vi "Main.vi"(11 "Module Admin":refnum<class "Delacor_lib_QMH_Module Admin.lvclass">) -> ()   [LabVIEW 2020, in "Launcher.lvlib"]
doc: "This template is based off of the Queued Message Handler design pattern and the Queued Message Handler project template that ships with LabVIEW.\n\nThe main difference is that the queue is private to this module and communication between modules is performed via Broadcast and Request events.\n\nRequest events are wrapped in public API methods and are handled in the Event Handling Loop (EHL) of this VI. Any module can register for Broadcast events sent by this module. The EHL generates messages based on user interface actions.\n\nThe Message Handling Loop (MHL) processes messages generated by the EHL, or by other messages. The messages are string values, so new messages can be added easily to the Message Cases case structure in the MHL. Each message cluster can also provide an optional value for Message Data, which is a variant that can be converted to whatever message-specific data is required.\n_____\nBased on Delacor QMH Project Template 5.0.0.82."
uses:
  Launcher.lvlib
  <vilib>/Delacor/Delacor QMH/Libraries/Module Admin_class/Delacor_lib_QMH_Module Admin.lvclass
  Module Data--cluster.ctl
  Stop Argument--cluster.ctl
  <vilib>/Delacor/Delacor QMH/Libraries/Message Queue_class/Delacor_lib_QMH_Message Queue.lvclass/Delacor_lib_QMH_Message Queue.ctl
  <vilib>/Delacor/Delacor QMH/Libraries/Module Admin_class/Delacor_lib_QMH_Module Admin.lvclass/Delacor_lib_QMH_Module Admin.ctl
  NXP LPCXpresso54608/NXP LPCXpresso54608.lvclass
  NXP LPCXpresso54608/NXP LPCXpresso54608.lvclass/NXP LPCXpresso54608.ctl
  Cypress CY8CKIT-059/Cypress CY8CKIT-059.lvclass
  Cypress CY8CKIT-059/Cypress CY8CKIT-059.lvclass/Cypress CY8CKIT-059.ctl
  Simulated Device/Simulated Device.lvclass
  <vilib>/Utility/miscctls.llb/LVPointTypeDef.ctl
  <vilib>/Delacor/Delacor QMH/Libraries/Message Queue_class/Delacor_lib_QMH_Enqueue Message (Single).vi
  <vilib>/Delacor/Delacor QMH/Libraries/Module Admin_class/Delacor_lib_QMH_Get External Launch.vi
  NXP LPCXpresso54608/Write Serial Port.vi
  Cypress CY8CKIT-059/Write Serial Port.vi
  <vilib>/Utility/error.llb/Error Cluster From Error Code.vi
  <vilib>/ErrorRing/Error Ring.xnode
  <vilib>/Delacor/Delacor QMH/Libraries/Message Queue_class/Delacor_lib_QMH_Message Queue.lvclass
  Hardware Interface/Hardware Interface.lvlib
panel:
  in  "Serial Port":refnum<visa-resource-name>
  in  "Device":enum16{"NXP", "Cypress", "Simulada"}(ring)
  in  "Open":bool
  out "error out":errorcluster
  out "Status":string
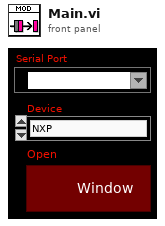
[diagram p1: front panel]
types:
  T1 = typedef "Launcher.lvlib/Request Events--cluster.ctl" = cluster{"Stop Module":refnum<user-event>, "Show Panel":refnum<user-event>, "Hide Panel":refnum<user-event>, "Get Module Execution Status":refnum<user-event>, "Show Diagram":refnum<user-event>}
  T2 = typedef "Hardware Interface.lvlib/Broadcast Events--cluster.ctl" = cluster{"Module Did Init":refnum<user-event>, "Status Updated":refnum<user-event>, "Error Reported":refnum<user-event>, "Module Did Stop":refnum<user-event>, "Update Module Execution Status":refnum<user-event>}
  T3 = typedef "Launcher.lvlib/Module Data--cluster.ctl" = cluster{"Status":string}
  T4 = enum32{"invalid lock state", "Not Locked", "Locked (No Password)", "Password-protected"}
  T5 = typedef "Launcher.lvlib/Stop Argument--cluster.ctl" = cluster{"Origin":string, "Exit via Stop Module Req?":bool, "Wait for Module to stop?":bool}
  T6 = typedef "LVPointTypeDef.ctl" = cluster{"Horizontal":i16, "Vertical":i16}
  T7 = enum32{"Invalid", "Standard", "Closed", "Hidden", "Minimized", "Maximized"}
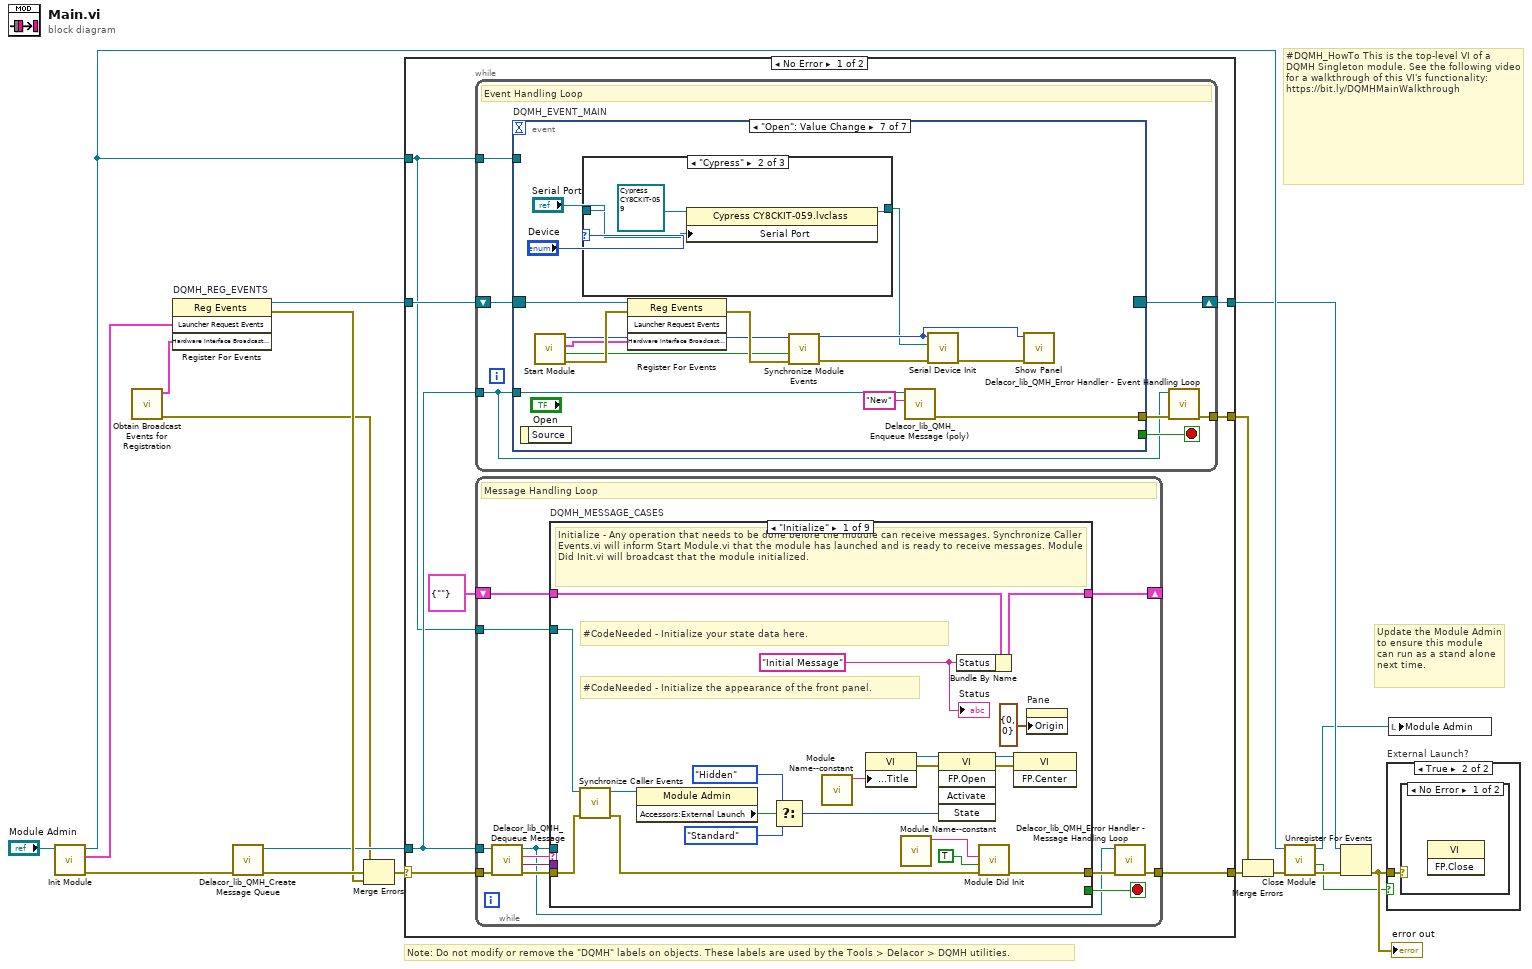
[diagram p0: block diagram]
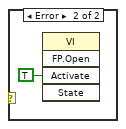
[diagram p3: hidden frame]
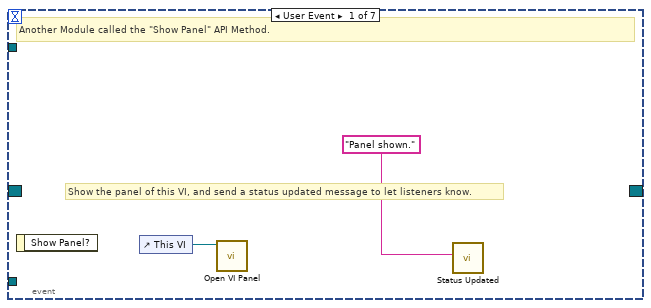
[diagram p4: hidden frame]
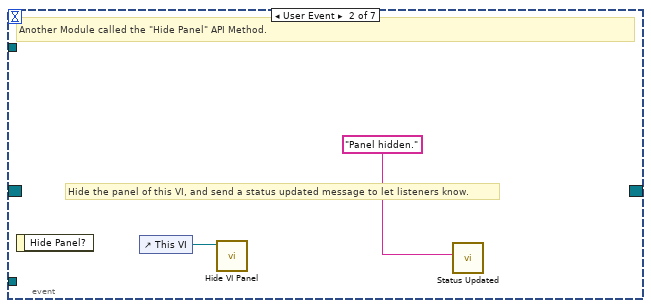
[diagram p5: hidden frame]
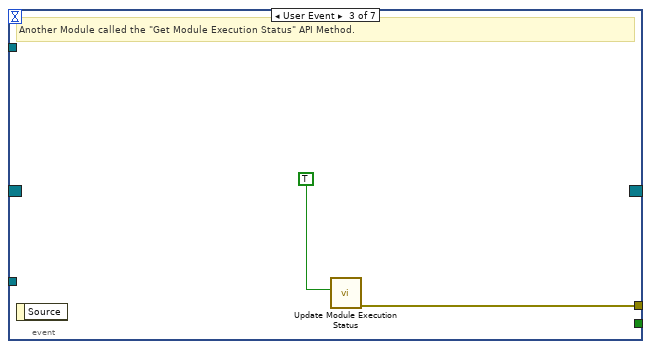
[diagram p6: hidden frame]
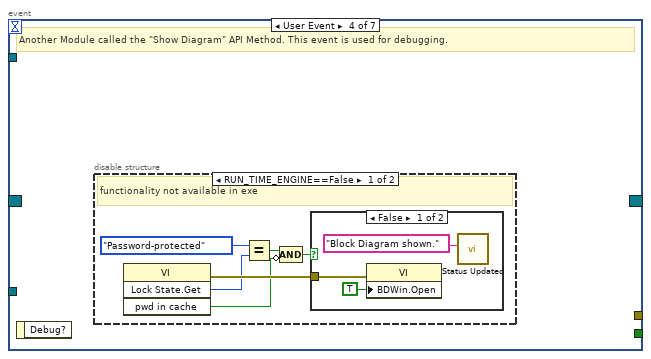
[diagram p7: hidden frame]
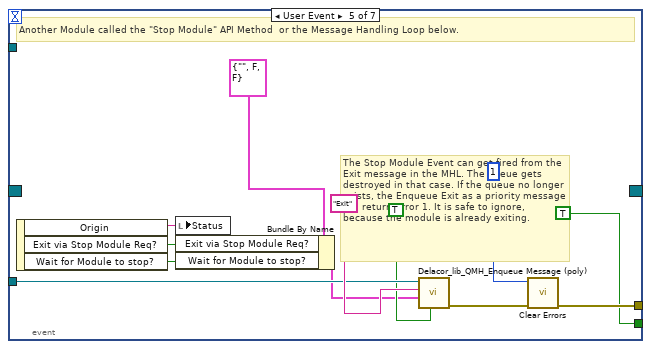
[diagram p10: hidden frame]
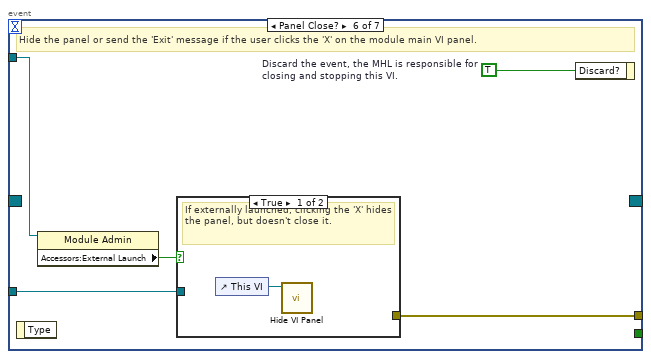
[diagram p11: hidden frame]
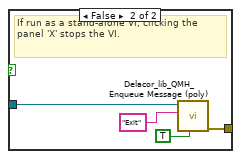
[diagram p12: hidden frame]
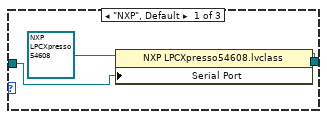
[diagram p13: hidden frame]
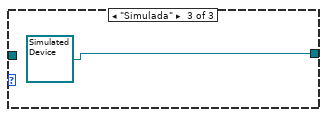
[diagram p14: hidden frame]
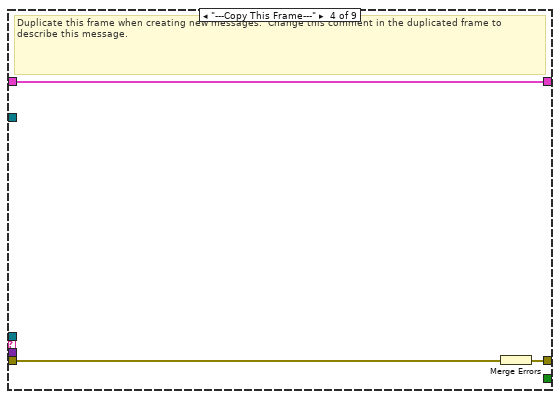
[diagram p17: hidden frame]
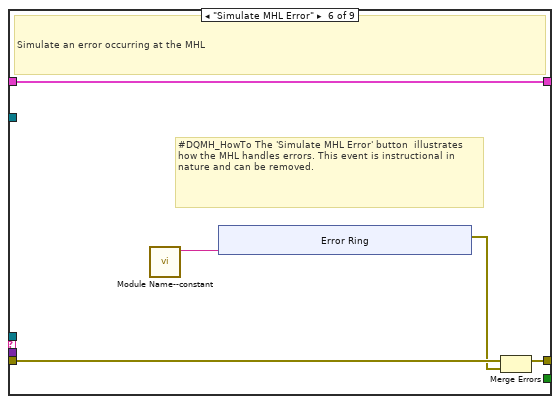
[diagram p19: hidden frame]
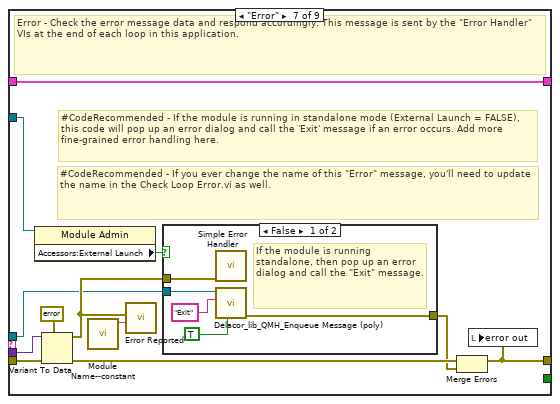
[diagram p20: hidden frame]
diagram:
  # "#DQMH_HowTo This is the top-level VI of a DQMH Singleton module. See the following video for a walkthrough of this VI's functionality: https://bit.ly/DQMHMainWalkthrough"
  # "Note: Do not modify or remove the \"DQMH\" labels on objects. These labels are used by the Tools > Delacor > DQMH utilities."
  # "Update the Module Admin to ensure this module can run as a stand alone next time."
  n1 = call "Init Module.vi"("Singleton Module Admin in"="Module Admin") -> ("error out"=w18:errorcluster, "Launcher Request Events"=w7:T1, "Singleton Module Admin out"=w10:refnum<class "Delacor_lib_QMH_Module Admin.lvclass">)  [unwired: 8 in]
  n2 = call "Obtain Broadcast Events for Registration.vi"() -> ("error out"=w1:errorcluster, "Hardware Interface Broadcast Events"=w2:T2)  [unwired: 9 in, 1 out]
  n3 = register-events "DQMH_REG_EVENTS"(w7, w2) -> (reference out=w8:refnum<event-registration>, error out=w11:errorcluster)  [unwired: 2 in]
  n4 = call <vilib>:"Delacor_lib_QMH_Create Message Queue.vi"("error in (no error)"=w18) -> ("error out"=w13:errorcluster, "Message Queue"=w6:refnum<class "Delacor_lib_QMH_Message Queue.lvclass">)  [unwired: 9 in]
  n5 = Merge Errors(w1, w13, w11) -> (w12:errorcluster)
  n6 = case shown="No Error" w12 {
    selector: w12 -> [w25 w195]
    tunnel: [w27 w194] -> w19
    tunnel: [w24 w200] -> w9
    tunnel: w8 -> [w22 w200]
    tunnel: w6 -> [w21 w193]
    tunnel: [w26 _] -> w16
    tunnel: w10 -> [w20 w196]
    frame No Error {
      n7 = while {
        tunnel: w21 -> [w28]
        shift-right: [w31] -> w24
        shift-left: w22 -> [w32]
        tunnel: [w33] -> w26
        tunnel: w20 -> [w29]
        stop <- w30 stop-if-true
        # "Event Handling Loop"
        n8 = event "DQMH_EVENT_MAIN" shown="[6] \"Open\": Value Change" {
          selector: w32 -> [_ _ _ _ _ _ w79]
          dyn-events: [_ _ _ _ _ _ _] -> w31
          timeout: _ -> [_ _ _ _ _ _ _]
          tunnel: [_ _ _ _ TRUE ("Discard?") _ _] -> w30
          tunnel: w28 -> [_ _ _ _ w57 w64 w85]
          tunnel: [_ _ w40 _ w60 w66 w86] -> w34
          tunnel: w29 -> [_ _ _ _ _ w63 _]
          event User Event {
            # "Show the panel of this VI, and send a status updated message to let listeners know."
            # "Another Module called the \"Show Panel\" API Method."
            n9 = event-data() -> ()  [unwired: 1 in, 1 out]
            n10 = control-ref of="This VI"() -> (w36:refnum<vi>)
            n11 = call "Open VI Panel.vi"("VI"=w36) -> ()  [unwired: 10 in, 1 out]
            n12 = call "Status Updated.vi"("Status"="Panel shown." ("format string")) -> ()  [unwired: 10 in, 1 out]
          }
          event User Event {
            # "Hide the panel of this VI, and send a status updated message to let listeners know."
            # "Another Module called the \"Hide Panel\" API Method."
            n13 = event-data() -> ()  [unwired: 1 in, 1 out]
            n14 = control-ref of="This VI"() -> (w38:refnum<vi>)
            n15 = call "Hide VI Panel.vi"("VI"=w38) -> ()  [unwired: 10 in, 1 out]
            n16 = call "Status Updated.vi"("Status"="Panel hidden." ("format string")) -> ()  [unwired: 10 in, 1 out]
          }
          event User Event {
            # "Another Module called the \"Get Module Execution Status\" API Method."
            n17 = event-data() -> ()  [unwired: 1 in, 1 out]
            n18 = call "Update Module Execution Status.vi"("Running?"=TRUE) -> ("error out"=w40:errorcluster)  [unwired: 10 in]
          }
          event User Event {
            # "Another Module called the \"Show Diagram\" API Method. This event is used for debugging."
            n19 = event-data() -> ()  [unwired: 1 in, 1 out]
            n20 = disable-structure shown="RUN_TIME_ENGINE==False" {
              frame condition #0 (active) {
                # "functionality not available in exe"
                n21 = invoke class="VI" method="Lock State.Get"() -> (error out=w46:errorcluster, "Get Lock State"=w45:T4, "pwd in cache"=w42:bool)  [unwired: 4 in, 1 out]
                n22 = Equal?(x=T4."Password-protected", y=w45) -> (x = y?=w43:bool)
                n23 = Compound Arithmetic op=AND(w43, invert w42) -> (w41:bool)
                n24 = case shown="False" w41 {
                  tunnel: w46 -> [w49 _]
                  frame False {
                    n25 = property class="VI"(error in=w49, "BDWin.Open"=TRUE ("Block Diagram Window:Open")) -> ()  [unwired: 1 in, 2 out]
                    n26 = call "Status Updated.vi"("Status"="Block Diagram shown." ("format string")) -> ()  [unwired: 10 in, 1 out]
                  }
                  frame True {
                    # "Password-protected VI, and the password is not in the cache. Do not show the diagram."
                  }
                }
              }
              frame condition #1 {
              }
            }
          }
          event User Event {
            # "The Stop Module Event can get fired from the Exit message in the MHL. The queue gets destroyed in that case. If the queue no longer exists, the Enqueue Exit as a priority message will return error 1. It is safe to ignore, because the module is already exiting."
            # "Another Module called the \"Stop Module\" API Method  or the Message Handling Loop below."
            n27 = event-data() -> ("Origin"=w56:string, "Exit via Stop Module Req?"=w52:bool, "Wait for Module to stop?"=w51:bool)  [unwired: 1 in]
            n28 = local write "Status"(w56) -> ()
            n29 = Bundle By Name(cluster=T5 {"Origin"="", "Exit via Stop Module Req?"=FALSE, "Wait for Module to stop?"=FALSE} ("Stop Argument"), "Exit via Stop Module Req?"=w52, "Wait for Module to stop?"=w51) -> (w50:T5)
            n30 = call-poly <vilib>:"Delacor_lib_QMH_Enqueue Message (poly).vi"("Priority Message? (F)"=TRUE, "Message Data"=w50, "Message"="Exit", "Message Queue in"=w57) -> ("error out"=w61:errorcluster)  [unwired: 6 in, 1 out]
            n31 = call <vilib>:"Clear Errors.vi"("error in (no error)"=w61, "specific error code to clear (0: all)"=1) -> ("error out"=w60:errorcluster)  [unwired: 4 in, 1 out]
          }
          event Panel Close? {
            w65 = TRUE  # Discard the event, the MHL is responsible for closing and stopping this VI.
            # "Hide the panel or send the 'Exit' message if the user clicks the 'X' on the module main VI panel."
            n32 = event-data() -> ()  [unwired: 1 in, 1 out]
            n33 = property class="Module Admin"(reference=w63) -> ("Accessors:External Launch"=w62:bool)  [unwired: 1 in, 2 out]
            n34 = case shown="True" w62 {
              tunnel: w64 -> [_ w70]
              tunnel: [_ w71] -> w66
              frame True {
                # "If externally launched, clicking the 'X' hides the panel, but doesn't close it."
                n35 = control-ref of="This VI"() -> (w67:refnum<vi>)
                n36 = call "Hide VI Panel.vi"("VI"=w67) -> ()  [unwired: 10 in, 1 out]
              }
              frame False {
                # "If run as a stand-alone VI, clicking the panel 'X' stops the VI."
                n37 = call-poly <vilib>:"Delacor_lib_QMH_Enqueue Message (poly).vi"("Priority Message? (F)"=TRUE, "Message"="Exit", "Message Queue in"=w70) -> ("error out"=w71:errorcluster)  [unwired: 7 in, 1 out]
              }
            }
            n38 = event-data("Discard?"=w65) -> ()  [unwired: 1 in, 1 out]
          }
          event "Open": Value Change {
            n39 = event-data() -> ()  [unwired: 1 in, 1 out]
            n40 = call "Start Module.vi"() -> ("error out"=w82:errorcluster, "Wait for Event Sync?"=w80:bool, "Hardware Interface Broadcast Events"=w78:T2, "Module ID"=w81:i32)  [unwired: 8 in]
            n41 = case shown="\"Cypress\"" "Device" {
              tunnel: [w88 w92 refnum<class "Simulated Device.lvclass"> refnum ("Simulated Device.lvclass")] -> w72
              tunnel: "Serial Port" -> [w87 w90 _]
              frame "NXP", Default {
                n42 = property class="NXP LPCXpresso54608.lvclass"(reference=refnum<class "NXP LPCXpresso54608.lvclass"> refnum ("NXP LPCXpresso54608.lvclass"), "Serial Port"=w87) -> (reference out=w88:refnum<class "NXP LPCXpresso54608.lvclass">)  [unwired: 1 in, 1 out]
              }
              frame "Cypress" {
                n43 = property class="Cypress CY8CKIT-059.lvclass"(reference=refnum<class "Cypress CY8CKIT-059.lvclass"> refnum ("Cypress CY8CKIT-059.lvclass"), "Serial Port"=w90) -> (reference out=w92:refnum<class "Cypress CY8CKIT-059.lvclass">)  [unwired: 1 in, 1 out]
              }
              frame "Simulada" {
              }
            }
            n44 = register-events(reference=w79, error in=w82, w78) -> (error out=w83:errorcluster)  [unwired: 1 in, 1 out]
            n45 = call "Synchronize Module Events.vi"("error in (no error)"=w83, "Wait for Event Sync?"=w80, "Module ID"=w81) -> ("error out"=w77:errorcluster, "Module ID (dup)"=w75:i32)  [unwired: 7 in]
            n46 = call-poly <vilib>:"Delacor_lib_QMH_Enqueue Message (poly).vi"("Message"="New", "Message Queue in"=w85) -> ("error out"=w86:errorcluster)  [unwired: 8 in, 1 out]
            n47 = call "Serial Device Init.vi"("error in (no error)"=w77, "MCU.lvclass"=w72, "Module ID"=w75) -> ("error out"=w76:errorcluster)  [unwired: 8 in]
            n48 = call "Show Panel.vi"("error in (no error)"=w76, "Module ID"=w75) -> ()  [unwired: 9 in, 1 out]
          }
        }
        n49 = call-dynamic "Delacor_lib_QMH_Error Handler - Event Handling Loop.vi"("error in (no error)"=w34, "Message Queue in"=w28) -> ("dup error in"=w33:errorcluster)  [unwired: 8 in, 1 out]
      }
      n50 = while {
        tunnel: w21 -> [w96]
        shift-right: [w100] -> _
        shift-left: T3 {"Status"=""} ("Data Cluster") -> [w101]
        tunnel: w25 -> [w104]
        tunnel: [w102] -> w27
        tunnel: w20 -> [w94]
        stop <- w99 stop-if-true
        # "Message Handling Loop"
        n51 = call-dynamic "Delacor_lib_QMH_Dequeue Message.vi"("error in (no error)"=w104, "Message Queue in"=w96) -> ("error out"=w103:errorcluster, "Message Data"=w97:variant, "Message"=w98:string, "Message Queue out"=w95:refnum<class "Delacor_lib_QMH_Message Queue.lvclass">)  [unwired: 6 in]
        n52 = case "DQMH_MESSAGE_CASES" shown="\"Initialize\"" w98 {
          selector: w98 -> [_ _ _ _ _ _ _ _ w180]
          tunnel: w95 -> [_ _ _ _ _ _ w150 w172 _]
          tunnel: w103 -> [w123 w127 w129 w132 w134 w139 w157 w178 w182]
          tunnel: [w121 w127 w129 w131 w134 w138 w153 w175 w183] -> w105
          tunnel: w101 -> [w112 w126 w128 w130 w133 w136 w152 w171 w181]
          tunnel: [w111 w126 w128 w130 w133 w136 w152 w171 w181] -> w100
          tunnel: [_ _ _ _ _ _ _ w170 _] -> w99
          tunnel: w97 -> [_ _ _ _ _ _ w151 w169 _]
          tunnel: w94 -> [w113 _ _ _ _ _ w149 w164 _]
          frame "Initialize" {
            w106 = "Initial Message" ("Initial Message")
            # "#CodeNeeded - Initialize the appearance of the front panel."
            # "#CodeNeeded - Initialize your state data here."
            # "Initialize - Any operation that needs to be done before the module can receive messages. Synchronize Caller Events.vi will inform Start Module.vi that the module has launched and is ready to receive messages. Module Did Init.vi will broadcast that the module initialized."
            n53 = call "Synchronize Caller Events.vi"("error in (no error)"=w123, "Singleton Module Admin in"=w113) -> ("error out"=w122:errorcluster, "Singleton Module Admin out"=w108:refnum<class "Delacor_lib_QMH_Module Admin.lvclass">)  [unwired: 8 in]
            n54 = property class="Module Admin"(reference=w108) -> ("Accessors:External Launch"=w117:bool)  [unwired: 1 in, 2 out]
            n55 = Select(t=T7."Hidden" ("State"), s=w117, f=T7."Standard" ("State")) -> (s? t:f=w114:T7)
            n56 = call "Module Name--constant.vi"() -> ("Module Name"=w120:string)  [unwired: 11 in]
            n57 = property class="VI"("Front Panel.Title"=w120) -> (reference out=w119:refnum<vi>, error out=w125:errorcluster)  [unwired: 2 in]
            n58 = call "Module Name--constant.vi"() -> ("Module Name"=w109:string)  [unwired: 11 in]
            n59 = invoke class="VI" method="FP.Open"(reference=w119, error in=w125, "State"=w114) -> (reference out=w118:refnum<vi>, error out=w124:errorcluster)  [unwired: 2 in, 3 out]
            n60 = Bundle By Name(cluster=w112, "Status"=w106) -> (w111:T3)
            n61 = call "Module Did Init.vi"("error in (no error)"=w122, "Initialized?"=TRUE, "Origin"=w109) -> ("error out"=w121:errorcluster)  [unwired: 8 in]
            n62 = invoke class="VI" method="FP.Center"(reference=w118, error in=w124) -> ()  [unwired: 1 in, 3 out]
            n63 = property on="Pane" class="Pane"("Origin"=T6 {"Horizontal"=0, "Vertical"=0}) -> ()  [unwired: 2 in, 2 out]
            "Status" <- w106
          }
          frame "New" {
          }
          frame "--- Module Specific ---" {
            # "Separator -- The following cases handle messages specific to this Module."
          }
          frame "---Copy This Frame---" {
            # "Duplicate this frame when creating new messages.  Change this comment in the duplicated frame to describe this message."
            n64 = Merge Errors(w132) -> (w131:errorcluster)
          }
          frame "--- Exit and Error Handling---" {
            # "Separator - The following cases handle errors and exit messages."
          }
          frame "Simulate MHL Error" {
            # "#DQMH_HowTo The 'Simulate MHL Error' button  illustrates how the MHL handles errors. This event is instructional in nature and can be removed."
            # "Simulate an error occurring at the MHL"
            n65 = call "Module Name--constant.vi"() -> ("Module Name"=w135:string)  [unwired: 11 in]
            n66 = xnode "Error Ring"("parameter 0"=w135) -> ("error out"=w137:errorcluster)
            n67 = Merge Errors(w139, w137) -> (w138:errorcluster)
          }
          frame "Error" {
            # "#CodeRecommended - If you ever change the name of this \"Error\" message, you'll need to update the name in the Check Loop Error.vi as well."
            # "#CodeRecommended - If the module is running in standalone mode (External Launch = FALSE), this code will pop up an error dialog and call the 'Exit' message if an error occurs. Add more fine-grained error handling here."
            # "Error - Check the error message data and respond accordingly. This message is sent by the \"Error Handler\" VIs at the end of each loop in this application."
            n68 = property class="Module Admin"(reference=w149) -> ("Accessors:External Launch"=w148:bool)  [unwired: 1 in, 2 out]
            n69 = Variant To Data(error in=w157, type=errorcluster {"status"=FALSE, "code"=0, "source"=""} ("error constant"), Variant=w151) -> (data=w158:errorcluster, error out=w155:errorcluster)
            n70 = call "Module Name--constant.vi"() -> ("Module Name"=w147:string)  [unwired: 11 in]
            n71 = call "Error Reported.vi"("Additional Information"=w147, "Error"=w158) -> ()  [unwired: 9 in, 1 out]
            n72 = case shown="False" w148 {
              tunnel: [w163 _] -> w154
              tunnel: w150 -> [w161 _]
              tunnel: w158 -> [w162 _]
              frame False {
                # "If the module is running standalone, then pop up an error dialog and call the \"Exit\" message."
                n73 = call <vilib>:"Simple Error Handler.vi"("error in (no error)"=w162) -> ()  [unwired: 4 in, 5 out]
                n74 = call-poly <vilib>:"Delacor_lib_QMH_Enqueue Message (poly).vi"("Priority Message? (F)"=TRUE, "Message"="Exit", "Message Queue in"=w161) -> ("error out"=w163:errorcluster)  [unwired: 7 in, 1 out]
              }
              frame True {
                # "If the module was launched externally, calling the Error Reported broadcast VI is the only action performed by the \"Error\" message. The module's caller can then process the error appropriately."
              }
            }
            n75 = Merge Errors(w155, w154) -> (w153:errorcluster)
            n76 = local write "error out"(w153) -> ()
          }
          frame "Exit" {
            w168 = 91  # 91: not all Exit messages will have an argument
            w170 = TRUE  # Stop the VI
            # "Release the message queue reference"
            # "#CodeNeeded - Add any required cleanup code here"
            # "Exit - Exit the application."
            n77 = Variant To Data(error in=w178, type=T5 {"Origin"="", "Exit via Stop Module Req?"=FALSE, "Wait for Module to stop?"=FALSE} ("Stop Argument"), Variant=w169) -> (data=w166:T5, error out=w174:errorcluster)
            n78 = call <vilib>:"Clear Errors.vi"("error in (no error)"=w174, "specific error code to clear (0: all)"=w168) -> ("error out"=w177:errorcluster)  [unwired: 4 in, 1 out]
            n79 = control-ref of="This VI"() -> (w165:refnum<vi>)
            n80 = call-dynamic "Delacor_lib_QMH_Release Message Queue.vi"("error in (no error)"=w177, "Message Queue"=w172) -> ("error out"=w176:errorcluster)  [unwired: 9 in]
            n81 = call "Handle Exit.vi"("Stop Argument"=w166, "Admin in"=w164, "VI reference"=w165) -> ("error out"=w173:errorcluster)  [unwired: 7 in, 1 out]
            n82 = Merge Errors(w176, w173) -> (w175:errorcluster)
          }
          frame Default {
            # "'Default' case only runs if there is a message that isn't defined in any of the other cases.  Output a programming error."
            n83 = call "Module Name--constant.vi"() -> ("Module Name"=w179:string)  [unwired: 11 in]
            n84 = xnode "Error Ring"("parameter 0"=w180, "parameter 1"=w179) -> ("error out"=w184:errorcluster)
            n85 = Merge Errors(w182, w184) -> (w183:errorcluster)
          }
        }
        n86 = call-dynamic "Delacor_lib_QMH_Error Handler - Message Handling Loop.vi"("error in (no error)"=w105, "Message Queue in"=w95) -> ("dup error in"=w102:errorcluster)  [unwired: 8 in, 1 out]
      }
    }
    frame Error {
      # "Synchronize Caller Events.vi will inform Start Module.vi that the module has launched and will let the code calling Start Module.vi register for broadcasts and would permit the caller receive the broadcast that an error occurred at launch time."
      n87 = call-dynamic "Delacor_lib_QMH_Release Message Queue.vi"("error in (no error)"=w195, "Message Queue"=w193) -> ("error out"=w194:errorcluster)  [unwired: 9 in]
      n88 = call "Synchronize Caller Events.vi"("Singleton Module Admin in"=w196) -> ("error out"=w201:errorcluster)  [unwired: 9 in, 1 out]
      n89 = call "Module Name--constant.vi"() -> ("Module Name"=w199:string)  [unwired: 11 in]
      n90 = Format Into String(format string="An error occurred during initialization. %s is no longer running.", w199) -> (resulting string=w197:string)  [unwired: 2 in, 1 out]
      n91 = Merge Errors(w194, w201) -> (w202:errorcluster)
      n92 = call "Error Reported.vi"("Additional Information"=w197, "Error"=w202) -> ()  [unwired: 9 in, 1 out]
    }
  }
  n93 = Merge Errors(w16, w19) -> (w15:errorcluster)
  n94 = call "Close Module.vi"("error in (no error)"=w15, "Module Admin in"=w10) -> ("error out"=w17:errorcluster, "External Launch"=w3:bool, "Module Admin out"=w4:refnum<class "Delacor_lib_QMH_Module Admin.lvclass">)  [unwired: 7 in]
  n95 = Unregister For Events(event registration refnum=w9, error in=w17) -> (error out=w14:errorcluster)
  "error out" <- w14
  n96 = case "External Launch?" shown="True" w3 {
    tunnel: w14 -> [_ w203]
    frame False {
    }
    frame True {
      n97 = case shown="No Error" w203 {
        frame No Error {
          n98 = invoke class="VI" method="FP.Close"() -> ()  [unwired: 3 in, 3 out]
        }
        frame Error {
          n99 = invoke class="VI" method="FP.Open"("Activate"=TRUE ("Activate?")) -> ()  [unwired: 4 in, 5 out]
        }
      }
    }
  }
  n100 = local write "Module Admin"(w4) -> ()
